vi "Build Default Name.vi"(3 "List of calibrations":refnum<vi>) -> (1 "Default name":string)   [LabVIEW 2009]
panel:
  # "Guillaume Plateau - yguig2@yahoo.fr"
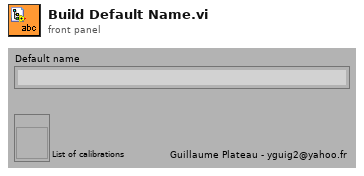
[diagram p1: front panel]
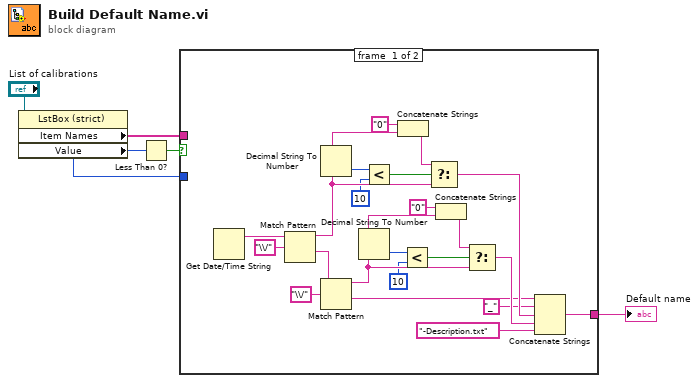
[diagram p0: block diagram]
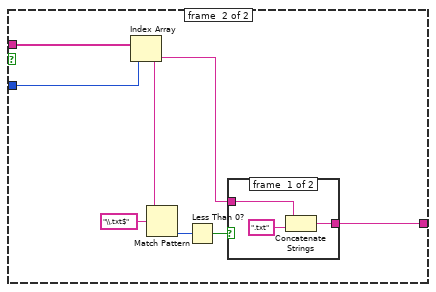
[diagram p2: hidden frame]
diagram:
  n1 = property class="LstBox (strict)"(reference="List of calibrations") -> ("Item Names"=w2:string[], "Value"=w1:i32)  [unwired: 1 in, 2 out]
  n2 = Less Than 0?(x=w1) -> (x < 0?=w4:bool)
  n3 = case shown="False" w4 {
    tunnel: [w27 w34] -> w5
    tunnel: w2 -> [_ w33]
    tunnel: w1 -> [_ w32]
    frame #0 {
      n4 = Get Date/Time String() -> (date string=w7:string)  [unwired: 3 in, 1 out]
      n5 = Match Pattern(string=w7, regular expression="\\/") -> (before substring=w18:string, after substring=w10:string)  [unwired: 1 in, 2 out]
      n6 = Decimal String To Number(string=w18) -> (number=w13:i32)  [unwired: 2 in, 1 out]
      n7 = Match Pattern(string=w10, regular expression="\\/") -> (before substring=w24:string, after substring=w11:string)  [unwired: 1 in, 2 out]
      n8 = Decimal String To Number(string=w24) -> (number=w23:i32)  [unwired: 2 in, 1 out]
      n9 = Less?(x=w13, y=10) -> (x < y?=w15:bool)
      n10 = Concatenate Strings("0" ("string"), w18) -> (w17:string)
      n11 = Less?(x=w23, y=10) -> (x < y?=w21:bool)
      n12 = Select(t=w17, s=w15, f=w18) -> (s? t:f=w25:string)
      n13 = Concatenate Strings("0" ("string"), w24) -> (w19:string)
      n14 = Select(t=w19, s=w21, f=w24) -> (s? t:f=w26:string)
      n15 = Concatenate Strings(w11, "_" ("string"), w25, w26, "-Description.txt" ("string")) -> (w27:string)
    }
    frame #1 {
      n16 = Index Array(array=w33, index=w32) -> (element=w30:string)
      n17 = Match Pattern(string=w30, regular expression="\\.txt$") -> (offset past match=w28:i32)  [unwired: 1 in, 3 out]
      n18 = Less Than 0?(x=w28) -> (x < 0?=w29:bool)
      n19 = case shown="True" w29 {
        tunnel: [w37 w38] -> w34
        tunnel: w30 -> [w35 w38]
        frame #0 {
          n20 = Concatenate Strings(w35, ".txt" ("string")) -> (w37:string)
        }
        frame #1 {
        }
      }
    }
  }
  "Default name" <- w5
